vi "Scripting_GetLibraryOfVI.vi"(8 "error in (no error)":errorcluster, 11 "VI in":refnum<vi>) -> (0 "error out":errorcluster, 1 "NotBelongingToLibrary":bool, 2 "Path":path, 3 "VI out":refnum<vi>, 4 "Name":string)   [LabVIEW 2020]
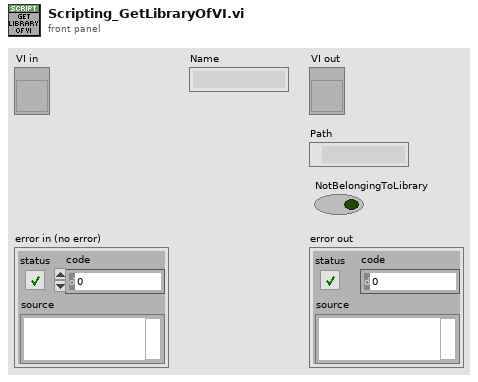
[diagram p1: front panel]
types:
  T1 = enum16{"Get Library Info", "Create Library Info", "Clear Library Info"}
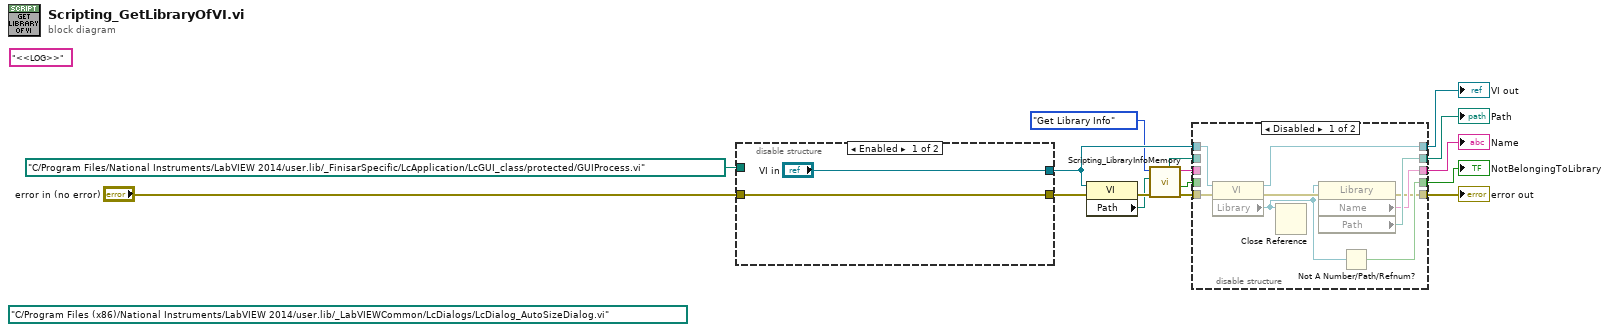
[diagram p0: block diagram]
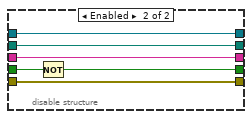
[diagram p2: hidden frame]
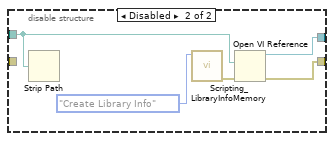
[diagram p3: hidden frame]
diagram:
  (unwired) "<<LOG>>" ("Name")
  (unwired) path "C:/Program Files (x86)/National Instruments/LabVIEW 2014/user.lib/_LabVIEWCommon/LcDialogs/LcDialog_AutoSizeDialog.vi"
  n1 = disable-structure shown="Enabled" {
    disable-tunnel: ["VI in" w23] -> w14
    disable-tunnel: path "C:/Program Files/National Instruments/LabVIEW 2014/user.lib/_FinisarSpecific/LcApplication/LcGUI_class/protected/GUIProcess.vi" -> [_ w21]
    disable-tunnel: [w17 w22] -> w10
    disable-tunnel: "error in (no error)" -> [w17 _]
    frame Enabled {
    }
    frame Disabled {
      n2 = Strip Path(path=w21) -> ()  [unwired: 2 out]
      n3 = call "Scripting_LibraryInfoMemory.vi"("Action"=T1."Create Library Info") -> ("error out"=w20:errorcluster)  [unwired: 6 in, 4 out]
      n4 = Open VI Reference(vi path=w21, error in (no error)=w20) -> (vi reference=w23:refnum<vi>, error out=w22:errorcluster)  [unwired: 4 in]
    }
  }
  n5 = property class="VI"(reference=w14, error in=w10) -> (error out=w7:errorcluster, "Path"=w5:path)  [unwired: 1 out]
  n6 = call "Scripting_LibraryInfoMemory.vi"("error in (no error)"=w7, "ViPath"=w5, "Action"=T1."Get Library Info") -> ("error out"=w1:errorcluster, "Found"=w2:bool, "LibraryName"=w4:string, "LibaryPath"=w3:path)  [unwired: 4 in, 1 out]
  n7 = disable-structure shown="Disabled" {
    disable-tunnel: [w32 w37] -> w16
    disable-tunnel: [w31 w38] -> w15
    disable-tunnel: w14 -> [w30 w33]
    disable-tunnel: [w29 w33] -> w13
    disable-tunnel: [w28 w35] -> w12
    disable-tunnel: w1 -> [w27 w34]
    disable-tunnel: [w26 w34] -> w9
    disable-tunnel: w4 -> [_ w38]
    disable-tunnel: w3 -> [_ w37]
    disable-tunnel: w2 -> [_ w36]
    frame Disabled {
      n8 = property class="VI"(reference=w30, error in=w27) -> (reference out=w29:refnum<vi>, error out=w25:errorcluster, "Library"=w24:refnum<vi>)
      n9 = Close Reference(reference=w24) -> ()  [unwired: 1 in, 1 out]
      n10 = property class="Library"(reference=w24, error in=w25) -> (error out=w26:errorcluster, "Name"=w31:string, "Path"=w32:path)  [unwired: 1 out]
      n11 = Not A Number/Path/Refnum?(number/path/refnum=w24) -> (NaN/Path/Refnum?=w28:bool)
    }
    frame Enabled {
      n12 = Not(x=w36) -> (.not. x?=w35:bool)
    }
  }
  "Path" <- w16
  "Name" <- w15
  "error out" <- w9
  "VI out" <- w13
  "NotBelongingToLibrary" <- w12
